vi "FrequencyToMillisecondsWithDefault.vi"(10 "Frequency":dbl, 11 "Default in":i64) -> (3 "Default out":i64)   [LabVIEW 2018, in "ScratchpadLibrary.lvlib"]
uses:
  Scratchpad/ScratchpadLibrary.lvlib
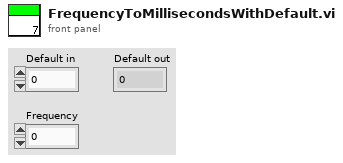
[diagram p1: front panel]
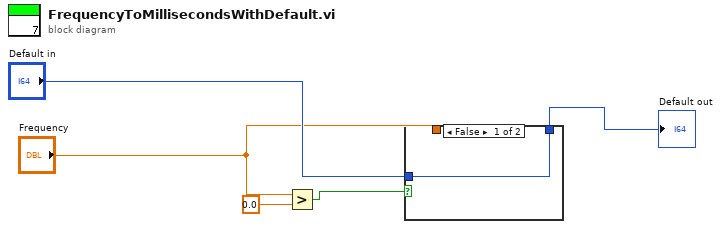
[diagram p0: block diagram]
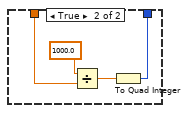
[diagram p2: hidden frame]
diagram:
  n1 = Greater?(x="Frequency", y=0.0) -> (0:w2:bool)
  n2 = case shown="False" w2 {
    tunnel: [w6 w9] -> w4
    tunnel: "Frequency" -> [_ w8]
    tunnel: "Default in" -> [w6 _]
    frame False {
    }
    frame True {
      n3 = Divide(x=1000.0, y=w8) -> (x/y=w10:dbl)
      n4 = To Quad Integer(1:w10) -> (0:w9:i64)
    }
  }
  "Default out" <- w4
